vi "Acquisition_1s.vi"(0 "connection ID":refnum<k5>, 1 "File ACQ data":path=path "C:/VIPlabview/Files/ACQbinaryData.dat", 5 "LayerID":u32=65535 format="%x", 7 "ChipID":u32=65535 format="%x", 9 "ACQ parameters":u32[](array[numeric])=[2, 0, 39999, 1000], 11 "error in (no error)":errorcluster, 12 "Acquisition time (s)":u32=5) -> (4 "connection ID out":refnum<k5>, 8 "Events":u32, 10 "ACQ WatchDog timeout":bool, 14 "Answer":string, 15 "error out":errorcluster)   [LabVIEW 2015, in "VIPM2.lvlib"]
doc: "<b>Es mostra el Front Panel en la crida !!!!!</b>\ncentrat i de mida fixa."
uses:
  VIPM2.lvlib
panel:
  out "Actual time":dbl
  in  "STOP ACQ":bool
  out "Ready to receive parameters":string
  # "Acquisition in progress"
  # "Stop Acquisition"
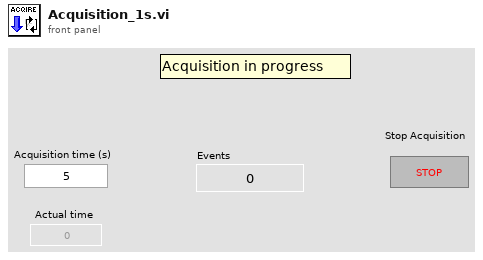
[diagram p1: front panel]
types:
  T1 = enum16{"open", "replace", "create", "open or create", "replace or create", "replace or create with confirmation"}
  T2 = enum16{"Standard", "Buffered", "CRLF", "Immediate"}
  T3 = enum16{"big-endian, network order", "native, host order", "little-endian"}
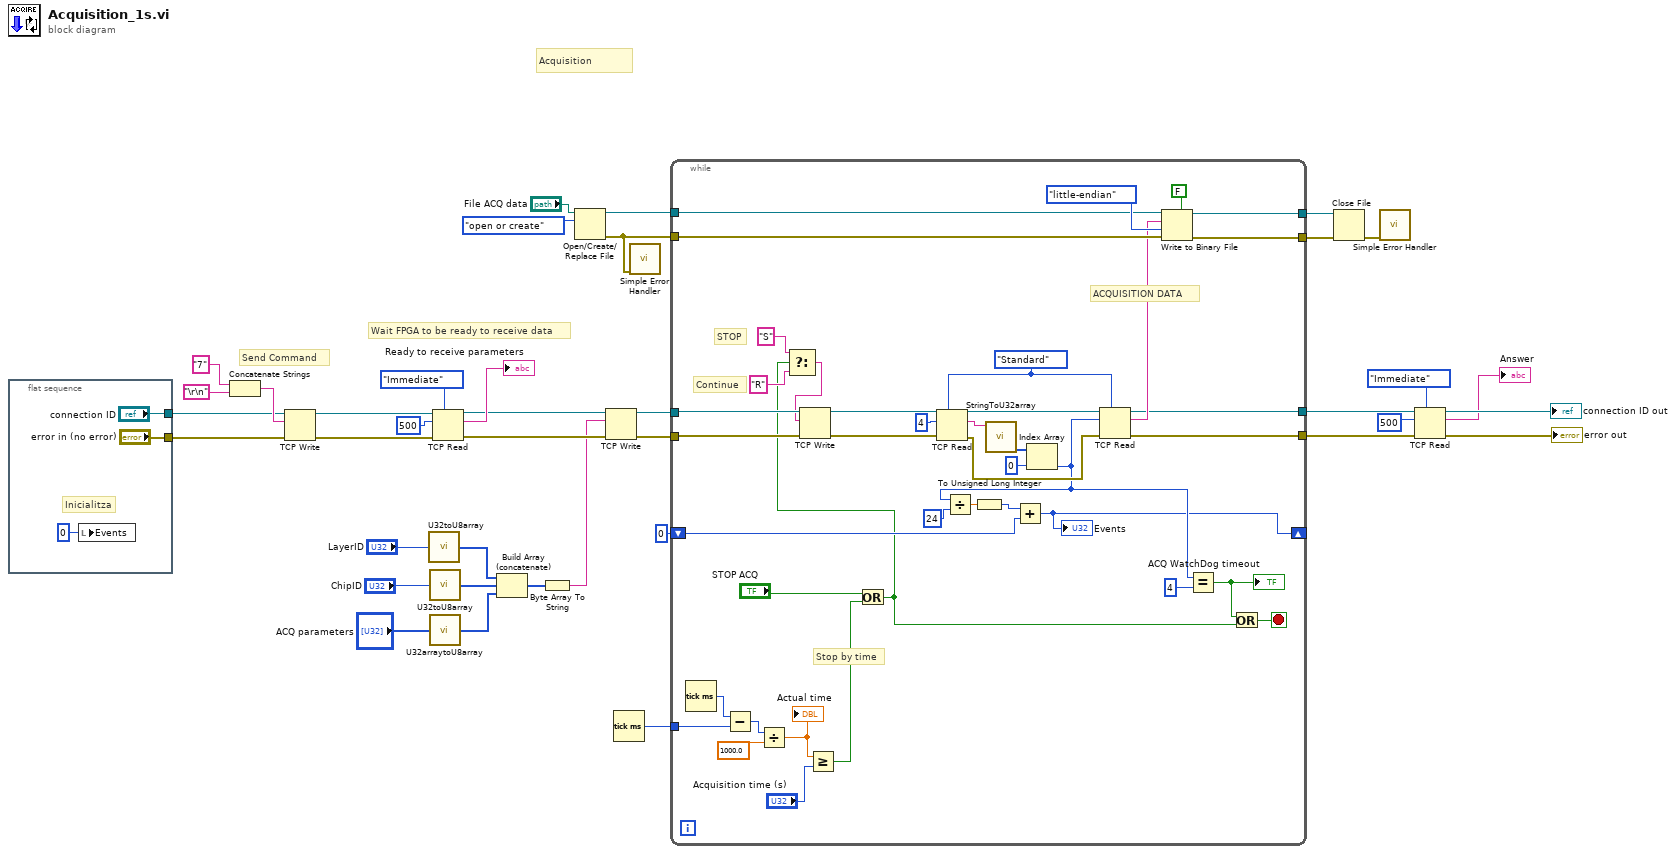
[diagram p0: block diagram]
diagram:
  # "Wait FPGA to be ready to receive data"
  # "Send Command"
  # "Acquisition"
  n1 = flat-sequence {
    tunnel: ["error in (no error)"] -> w35
    tunnel: ["connection ID"] -> w34
    frame #0 {
      # "Inicialitza"
      n2 = local write "Events"(u32 0 ("Events")) -> ()
    }
  }
  n3 = Concatenate Strings("7" ("string"), "\r\n") -> (w36:string)
  n4 = TCP Write(connection ID=w34, data in=w36, error in (no error)=w35) -> (connection ID out=w30:refnum<k5>, error out=w29:errorcluster)  [unwired: 1 in, 1 out]
  n5 = call "U32toU8array.vi"("x"="LayerID") -> ("ArrayU8"=w18:u8[])
  n6 = call "U32toU8array.vi"("x"="ChipID") -> ("ArrayU8"=w16:u8[])
  n7 = call "U32arraytoU8array.vi"("ArrayU32"="ACQ parameters") -> ("ArrayU8"=w14:u8[])
  n8 = TCP Read(connection ID=w30, bytes to read=500, error in (no error)=w29, 7:T2."Immediate" ("mode (standard)")) -> (connection ID out=w27:refnum<k5>, data out=→"Ready to receive parameters":string, error out=w26:errorcluster)  [unwired: 1 in]
  n9 = Build Array (concatenate)(w18, w16, w14) -> (w19:u8[])
  n10 = Byte Array To String(unsigned byte array=w19) -> (string=w25:string)
  n11 = Open/Create/Replace File(file path (use dialog)="File ACQ data", operation (0:open)=T1."open or create") -> (refnum out=w8:refnum<file>, error out=w7:errorcluster)  [unwired: 4 in, 1 out]
  n12 = TCP Write(connection ID=w27, data in=w25, error in (no error)=w26) -> (connection ID out=w13:refnum<k5>, error out=w12:errorcluster)  [unwired: 1 in, 1 out]
  n13 = Tick Count (ms)() -> (millisecond timer value=w1:u32)
  n14 = call <vilib>:"Simple Error Handler.vi"("error in (no error)"=w7) -> ()  [unwired: 4 in, 5 out]
  n15 = while {
    tunnel: w13 -> [w80]
    tunnel: w12 -> [w79]
    shift-right: [w62] -> _
    shift-left: u32 0 -> [w63]
    tunnel: w7 -> [w58]
    tunnel: w8 -> [w59]
    tunnel: [w56] -> w6
    tunnel: [w55] -> w5
    tunnel: [w54] -> w4
    tunnel: [w53] -> w3
    tunnel: w1 -> [w46]
    stop <- w52 stop-if-true
    w75 = T2."Standard" ("mode (standard)")
    # "Stop by time"
    # "ACQUISITION DATA"
    # "Continue"
    # "STOP"
    n16 = Tick Count (ms)() -> (millisecond timer value=w47:u32)
    n17 = Subtract(x=w47, y=w46) -> (x-y=w45:u32)
    n18 = Divide(x=w45, y=1000.0) -> (x/y=w44:dbl)
    "Actual time" <- w44
    n19 = Greater Or Equal?(x=w44, y="Acquisition time (s)") -> (x >= y?=w42:bool)
    n20 = Or(x="STOP ACQ", y=w42) -> (x .or. y?=w49:bool)
    n21 = Select(t="S" ("string"), s=w49, f="R" ("string")) -> (s? t:f=w78:string)
    n22 = TCP Write(connection ID=w80, data in=w78, error in (no error)=w79) -> (connection ID out=w68:refnum<k5>, error out=w67:errorcluster)  [unwired: 1 in, 1 out]
    n23 = TCP Read(connection ID=w68, bytes to read=4, error in (no error)=w67, 7:w75) -> (connection ID out=w73:refnum<k5>, data out=w66:string, error out=w74:errorcluster)  [unwired: 1 in]
    n24 = call "StringToU32array.vi"("String"=w66) -> ("U32array"=w65:u32[])  [unwired: 2 out]
    n25 = Index Array(array=w65, index=0) -> (element=w64:u32)
    n26 = Divide(x=w64, y=u32 24) -> (x/y=w70:dbl)
    n27 = To Unsigned Long Integer(number=w70) -> (unsigned 32bit integer=w69:u32)
    n28 = Add(x=w69, y=w63) -> (x+y=w62:u32)
    "Events" <- w62
    n29 = TCP Read(connection ID=w73, bytes to read=w64, error in (no error)=w74, 7:w75) -> (connection ID out=w55:refnum<k5>, data out=w57:string, error out=w56:errorcluster)  [unwired: 1 in]
    n30 = Write to Binary File(file (use dialog)=w59, data=w57, error in=w58, 5:FALSE ("prepend array or string size? (T)"), 9:T3."little-endian" ("byte order (0:big-endian, network order)")) -> (refnum out=w54:refnum<file>, error out=w53:errorcluster)  [unwired: 1 in, 1 out]
    n31 = Equal?(x=w64, y=u32 4) -> (x = y?=w51:bool)
    "ACQ WatchDog timeout" <- w51
    n32 = Or(x=w51, y=w49) -> (x .or. y?=w52:bool)
  }
  n33 = Close File(refnum=w4, error in=w3) -> (error out=w2:errorcluster)  [unwired: 1 out]
  n34 = call <vilib>:"Simple Error Handler.vi"("error in (no error)"=w2) -> ()  [unwired: 4 in, 5 out]
  n35 = TCP Read(connection ID=w5, bytes to read=500, error in (no error)=w6, 7:T2."Immediate" ("mode (standard)")) -> (connection ID out=→"connection ID out":refnum<k5>, data out=→"Answer":string, error out=→"error out":errorcluster)  [unwired: 1 in]
